vi "global variable.vi"() -> ()   [LabVIEW 2017]
panel:
  out "left arm distance":dbl
  out "leftarmforward":dbl[](array[numeric])
  out "newed":dbl
  out "gripper":dbl[](array[numeric])
  out "LA position":dbl
  out "j 3":dbl[](array[numeric])
  out "joint positions 2":dbl[](array[numeric])
  out "joint positions1":dbl[](array[numeric])
  out "11,10,9.6":dbl[](array[numeric])
  out "stringfromp":string
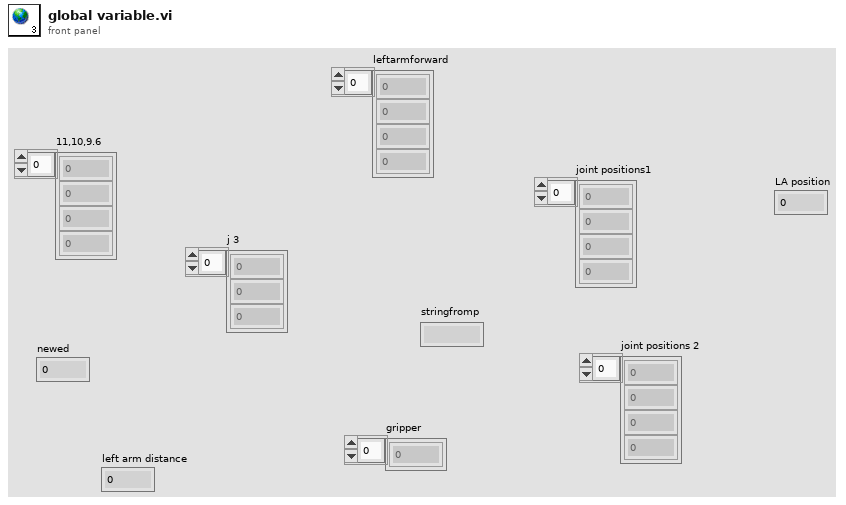
[diagram p1: front panel]
diagram:
